vi "write analog tasks.vi"(8 "error in (no error)":errorcluster, 11 "Waveform in":refnum<class "Waveform.lvclass">) -> (0 "error out":errorcluster, 3 "Waveform out":refnum<class "Waveform.lvclass">)   [LabVIEW 2012, in "Waveform.lvclass"]
uses:
  Waveform.lvclass
  <vilib>/DAQmx/write.llb/DAQmx Write (Analog Wfm 1Chan NSamp).vi
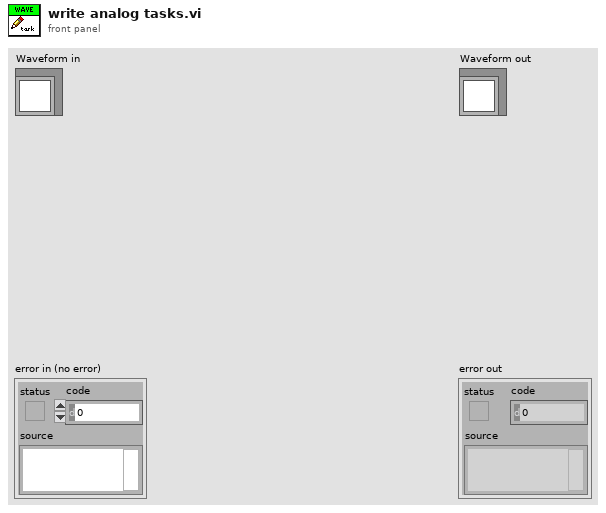
[diagram p1: front panel]
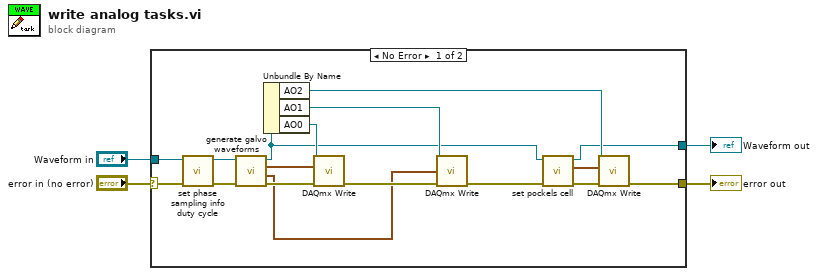
[diagram p0: block diagram]
diagram:
  n1 = case shown="No Error" "error in (no error)" {
    selector: "error in (no error)" -> [w18 w23]
    tunnel: [w9 w23] -> w3
    tunnel: [w5 w22] -> w1
    tunnel: "Waveform in" -> [w15 w22]
    frame No Error {
      n2 = call-dynamic "set phase sampling info duty cycle.vi"("error in (no error)"=w18, "Waveform in"=w15) -> ("error out"=w19:errorcluster, "Waveform out"=w16:refnum<class "Waveform.lvclass">)  [unwired: 8 in]
      n3 = call-dynamic "generate galvo waveforms.vi"("error in (no error)"=w19, "Waveform in"=w16) -> ("error out"=w17:errorcluster, "Waveform 2"=w13:waveform(dbl), "Waveform"=w14:waveform(dbl), "Waveform out"=w6:refnum<class "Waveform.lvclass">)  [unwired: 6 in]
      n4 = Unbundle By Name(w6) -> ("AO2"=w7:refnum<k21>, "AO1"=w12:refnum<k21>, "AO0"=w20:refnum<k21>)
      n5 = call-poly <vilib>:"DAQmx Write.vi"("task/channels in"=w20, "data"=w14, "error in"=w17) -> ("error out"=w21:errorcluster)  [unwired: 10 in, 2 out]
      n6 = call-poly <vilib>:"DAQmx Write.vi"("task/channels in"=w12, "data"=w13, "error in"=w21) -> ("error out"=w11:errorcluster)  [unwired: 10 in, 2 out]
      n7 = call-dynamic "set pockels cell.vi"("error in (no error)"=w11, "Waveform in"=w6) -> ("error out"=w10:errorcluster, "output waveform"=w8:waveform(dbl), "Waveform out"=w5:refnum<class "Waveform.lvclass">)  [unwired: 7 in]
      n8 = call-poly <vilib>:"DAQmx Write.vi"("task/channels in"=w7, "data"=w8, "error in"=w10) -> ("error out"=w9:errorcluster)  [unwired: 10 in, 2 out]
    }
    frame Error {
    }
  }
  "error out" <- w3
  "Waveform out" <- w1
